vi "measurement residual.vi"(10 "x_k|k-1":T1, 11 "z_k":T1) -> (3 "y~_k":T1)   [LabVIEW 2018]
uses:
  <vilib>/Analysis/Matrix/Datatypes/RealMatrix.ctl
  <vilib>/Analysis/Matrix/Numeric/Multiply/Multiply - RM,RM.vi
  <vilib>/Analysis/Matrix/Numeric/Subtract/Subtract - RM,RM.vi
  <vilib>/Analysis/Matrix/Numeric/Conversions/Matrix To Array - RM.vi
  <vilib>/Analysis/Matrix/NI_Matrix.lvlib
panel:
  out "y~_k":dbl[][](array[numeric])
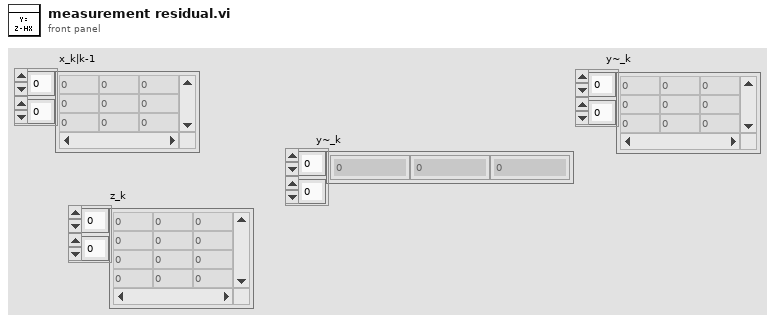
[diagram p1: front panel]
types:
  T1 = typedef "NI_Matrix.lvlib/RealMatrix.ctl" = dbl[][]
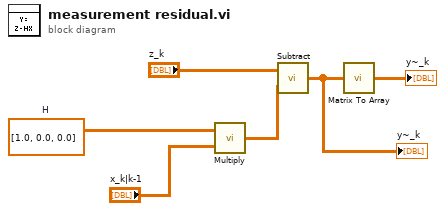
[diagram p0: block diagram]
diagram:
  w3 = T1 [[1.0, 0.0, 0.0]]  # H
  n1 = call-poly <vilib>:"Multiply.vi"("Real Matrix B"="x_k|k-1", "Real Matrix A"=w3) -> ("A * B"=w6:T1)
  n2 = call-poly <vilib>:"Subtract.vi"("Real Matrix B"=w6, "Real Matrix A"="z_k") -> ("A - B"=w2:T1)
  "y~_k" <- w2
  n3 = call-poly <vilib>:"Matrix To Array.vi"("Real Matrix"=w2) -> ("Real 2D Array"=→"y~_k":dbl[][])
